vi "CLSUIP_LocalizedStrings.vi"() -> ()   [LabVIEW 2020, in "MemberVICreation.lvlib"]
uses:
  <resource>/Framework/Providers/LVClassLibrary/NewAccessors/MemberVICreation.lvlib
panel:
  in  "no members":string="<No Data Members>"
  in  "Array Name <element>":string="%s <element>"
  in  "<class name> out":string="%s out"
  in  "<class name> in":string="%s in"
  in  "Read <element>.vi":string="Get %s.vi"
  in  "Write <element>.vi":string="Set %s.vi"
  in  "Element of <class name>":string="Element of %s"
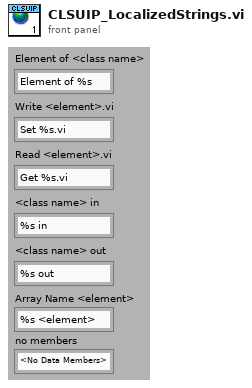
[diagram p1: front panel]
diagram:
